vi "Restore Configuration.vi"(8 "error in (no error)":errorcluster, 10 "File path":path, 11 "Measure Object in":refnum<class "NHMFL Synthesizer.lvclass">) -> (0 "error out":errorcluster, 1 "Section out":string, 2 "File path out":path, 3 "Measure Object out":refnum<class "NHMFL Synthesizer.lvclass">)   [LabVIEW 2018, in "NHMFL Synthesizer.lvclass"]
uses:
  NHMFL Synthesizer.lvclass
  Process Object/Process Object.lvclass
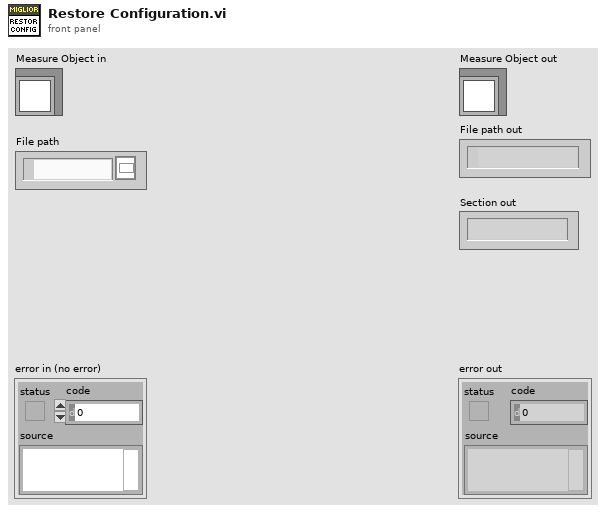
[diagram p1: front panel]
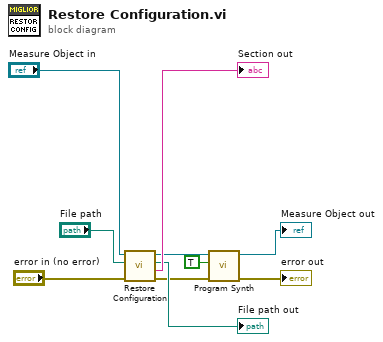
[diagram p0: block diagram]
diagram:
  n1 = call-parent "Restore Configuration.vi"("error in (no error)"="error in (no error)", "File path"="File path", "Measure Object in"="Measure Object in") -> ("error out"=w5:errorcluster, "Section out"=→"Section out":string, "File path out"=→"File path out":path, "Measure Object out"=w4:refnum<class "NHMFL Synthesizer.lvclass">)  [unwired: 5 in]
  n2 = call-dynamic "Program Synth.vi"("error in (no error)"=w5, "Check if valid device"=TRUE, "NHMFL Synthesizer in"=w4) -> ("error out"=→"error out":errorcluster, "NHMFL Synthesizer out"=→"Measure Object out":refnum<class "NHMFL Synthesizer.lvclass">)  [unwired: 7 in]
